vi "Tracer.vi"(8 "error in":errorcluster, 9 "Value":dbl, 10 "Operation Mode":enum16{"CC", "CV", "CR", "CW"}(ring), 11 "IT8800 Setting In In":T1={"VISA Resource Name"="", "Baud Rate"=19200, "Stop Bits"=20, "Wait For Read(ms)"=0, "Interface Type"=enum."VXI", "Limits"=[]} {"Stop Bits" items=["1.0"=10, "2.0"=20]; "Baud Rate" items=["2400"=2400, "4800"=4800, "9600"=9600, "19200"=19200]}) -> (0 "error out":errorcluster, 3 "IT8800 Setting In Out":T1={"VISA Resource Name"="", "Baud Rate"=19200, "Stop Bits"=20, "Wait For Read(ms)"=0, "Interface Type"=enum."VXI", "Limits"=[]} {"Stop Bits" items=["1.0"=10, "2.0"=20]; "Baud Rate" items=["2400"=2400, "4800"=4800, "9600"=9600, "19200"=19200]})   [LabVIEW 2018]
uses:
  Data Def/IT8800-Setting.ctl
  Data Def/IT8800-Operation Mode.ctl
  VI/IT8800-Configure Constant Current.vi
  VI/IT8800-Configure Constant Voltage.vi
  VI/IT8800-Configure Constant Power.vi
  VI/IT8800-Configure Constant Resistance.vi
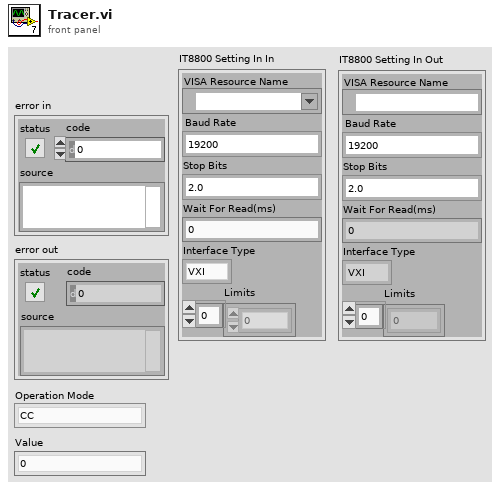
[diagram p1: front panel]
types:
  T1 = typedef "IT8800-Setting.ctl" = cluster{"VISA Resource Name":refnum<visa-resource-name>, "Baud Rate":u32, "Stop Bits":u16, "Wait For Read(ms)":u32, "Interface Type":enum16{"Unknow", "GPIB", "VXI", "GPIB-VXI", "Serial", "PXI", "TCPIP", "USB", "FireWire"}, "Limits":u16[]}
  T2 = typedef "IT8800-Operation Mode.ctl" = enum16{"Current", "Voltage", "Power", "Resistance"}
  T3 = typedef "IT8800-Measurement Data.ctl" = cluster{"Current (Amps)":dbl, "Power (Watts)":dbl, "Voltage (Volts)":dbl, "Elapsed Time (Sec) ":dbl}
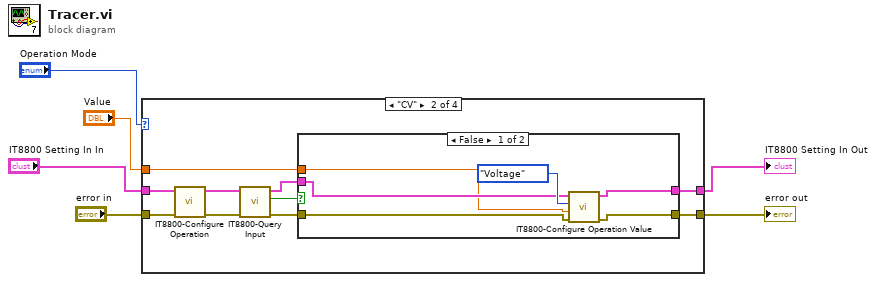
[diagram p0: block diagram]
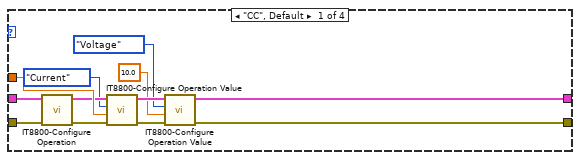
[diagram p2: hidden frame]
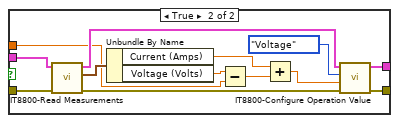
[diagram p3: hidden frame]
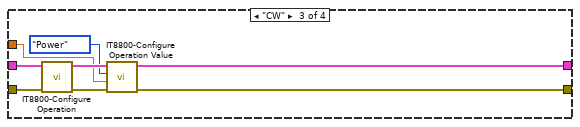
[diagram p4: hidden frame]
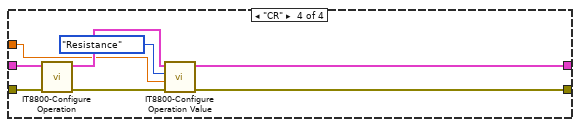
[diagram p5: hidden frame]
diagram:
  n1 = case shown="\"CV\"" "Operation Mode" {
    tunnel: "IT8800 Setting In In" -> [w12 w28 w55 w63]
    tunnel: "error in" -> [w10 w27 w54 w62]
    tunnel: "Value" -> [w18 w26 w49 w57]
    tunnel: [w14 w25 w52 w60] -> w2
    tunnel: [w15 w24 w51 w59] -> w1
    frame "CC", Default {
      n2 = call-poly "IT8800-Configure Operation.vi"("error in"=w10, "IT8800 Setting In In"=w12) -> ("error out"=w9:errorcluster, "IT8800 Setting In Out"=w11:T1)  [unwired: 8 in]
      n3 = call "IT8800-Configure Operation Value.vi"("error in"=w9, "Values (0)"=w18, "Value Type (0:Current)"=IT8800-Operation_Mode."Current", "IT8800 Setting In In"=w11) -> ("error out"=w16:errorcluster, "IT8800 Setting In Out"=w17:T1)  [unwired: 6 in]
      n4 = call "IT8800-Configure Operation Value.vi"("error in"=w16, "Values (0)"=10.0, "Value Type (0:Current)"=IT8800-Operation_Mode."Voltage", "IT8800 Setting In In"=w17) -> ("error out"=w15:errorcluster, "IT8800 Setting In Out"=w14:T1)  [unwired: 6 in]
    }
    frame "CV" {
      n5 = call-poly "IT8800-Configure Operation.vi"("error in"=w27, "IT8800 Setting In In"=w28) -> ("error out"=w23:errorcluster, "IT8800 Setting In Out"=w22:T1)  [unwired: 8 in]
      n6 = call "IT8800-Query Input.vi"("error in"=w23, "IT8800 Setting In In"=w22) -> ("error out"=w21:errorcluster, "Input?"=w19:bool, "IT8800 Setting In Out"=w20:T1)  [unwired: 7 in]
      n7 = case shown="False" w19 {
        tunnel: w26 -> [w29 w36]
        tunnel: [w32 w47] -> w25
        tunnel: [w30 w46] -> w24
        tunnel: w21 -> [w31 w44]
        tunnel: w20 -> [w33 w45]
        frame False {
          n8 = call "IT8800-Configure Operation Value.vi"("error in"=w31, "Values (0)"=w29, "Value Type (0:Current)"=IT8800-Operation_Mode."Voltage", "IT8800 Setting In In"=w33) -> ("error out"=w30:errorcluster, "IT8800 Setting In Out"=w32:T1)  [unwired: 6 in]
        }
        frame True {
          n9 = call "IT8800-Read Measurements.vi"("error in"=w44, "IT8800 Setting In In"=w45) -> ("error out"=w42:errorcluster, "Measurement Data"=w41:T3, "IT8800 Setting In Out"=w43:T1)  [unwired: 7 in]
          n10 = Unbundle By Name(w41) -> ("Current (Amps)"=w39:dbl, "Voltage (Volts)"=w40:dbl)
          n11 = Subtract(x=w40, y=w36) -> (x-y=w38:dbl)
          n12 = Add(x=w39, y=w38) -> (x+y=w35:dbl)
          n13 = call "IT8800-Configure Operation Value.vi"("error in"=w42, "Values (0)"=w35, "Value Type (0:Current)"=IT8800-Operation_Mode."Voltage", "IT8800 Setting In In"=w43) -> ("error out"=w46:errorcluster, "IT8800 Setting In Out"=w47:T1)  [unwired: 6 in]
        }
      }
    }
    frame "CW" {
      n14 = call-poly "IT8800-Configure Operation.vi"("error in"=w54, "IT8800 Setting In In"=w55) -> ("error out"=w50:errorcluster, "IT8800 Setting In Out"=w53:T1)  [unwired: 8 in]
      n15 = call "IT8800-Configure Operation Value.vi"("error in"=w50, "Values (0)"=w49, "Value Type (0:Current)"=IT8800-Operation_Mode."Power", "IT8800 Setting In In"=w53) -> ("error out"=w51:errorcluster, "IT8800 Setting In Out"=w52:T1)  [unwired: 6 in]
    }
    frame "CR" {
      n16 = call-poly "IT8800-Configure Operation.vi"("error in"=w62, "IT8800 Setting In In"=w63) -> ("error out"=w58:errorcluster, "IT8800 Setting In Out"=w61:T1)  [unwired: 8 in]
      n17 = call "IT8800-Configure Operation Value.vi"("error in"=w58, "Values (0)"=w57, "Value Type (0:Current)"=IT8800-Operation_Mode."Resistance", "IT8800 Setting In In"=w61) -> ("error out"=w59:errorcluster, "IT8800 Setting In Out"=w60:T1)  [unwired: 6 in]
    }
  }
  "error out" <- w1
  "IT8800 Setting In Out" <- w2
